vi "Double FFT Mesurament (Max Bin detection - Control - Init Wave&Window - Snapshot) test.vi"() -> ()   [LabVIEW 2014]
uses:
  <vilib>/Platform/TimedLoop/XDataNode/timing_clust.ctl
  <vilib>/Platform/TimedLoop/XDataNode/nitl_modes.ctl
  <vilib>/Platform/TimedLoop/XDataNode/wakeup.ctl
  <vilib>/rvi/Analysis/measure/FFT/simModelSupport/niFPGA FFT Streaming Sim Properties.ctl
  <vilib>/rvi/Analysis/measure/FFT/simModelSupport/niFPGA FFT Sim Stream Group Properties.ctl
  <vilib>/rvi/Analysis/measure/FFT/simModelSupport/niFPGA FFT Sim Types.ctl
  <vilib>/rvi/Analysis/measure/FFT/simModelSupport/niFpgaFFTSimArithmeticProperties.ctl
  <vilib>/rvi/Analysis/measure/FFT/simModelSupport/niFpgaFFTSimDfxp.ctl
  <vilib>/fxp/LVFixedPointQuantizationPolicyTypeDef.ctl
  <vilib>/rvi/Analysis/measure/FFT/XNode/niFpgaFFTButterflyDelays.ctl
  <vilib>/rvi/Emulation/niFpgaSctlEmulationGetInTimedLoop.vi
  <vilib>/rvi/Emulation/niFpgaEmulationReportErrorSimple.vi
  <vilib>/rvi/Emulation/niFpgaGetClockAttributes.vi
  <vilib>/rvi/Emulation/niFpgaCriticalErrorInLSC.vi
  <vilib>/rvi/Emulation/niFpgaEmulationIsFPGAContextNoSignature.vi
  <vilib>/rvi/errors/niFpgaSetErrorForExecOnDevCompSimple.vi
  <vilib>/rvi/eio/common/nirviEmuReportErrorAndStop.vi
  <vilib>/rvi/DataTransferAndStorage/Container/Common/niFpgaContainerGetUniqueNameForEmu.vi
  <vilib>/rvi/FIFO/Fifo_Resource/nirvififoEmulationSetSize.vi
  <vilib>/rvi/FIFO/Fifo_Resource/nirviFifoEmulationQueueMgr.vi
  <instcachedir>/0/nirviFifoEmulationQueueMgr_E5CAEC123FF24DC58D834DCA3CDAA9B5.lvgen/nirviFifoEmulationQueueMgr_E5CAEC123FF24DC58D834DCA3CDAA9B5_012.vi
  <vilib>/rvi/FIFO/Fifo_Resource/nirvififoEmulationCreateLock.vi
  <vilib>/rvi/Emulation/niFpgaProcessEmulError.vi
  <vilib>/rvi/FIFO/Fifo_Resource/nirvififoEmulationObtainLock.vi
  <vilib>/rvi/FIFO/Fifo_Resource/nirvififoEmulationReleaseLock.vi
  <vilib>/rvi/occurrence/nirviWaitOnOccurrenceBase.vi
  <vilib>/rvi/errors/nirviReportUnexpectedCaseInternalError.vi
  <vilib>/rvi/errors/nirviReportUnexpectedCaseInternalError (U32).vi
  <vilib>/rvi/Memory/Memory_Emulation/niFpgaMemoryEmulationCacheClearOnFirstRun.vi
  <vilib>/rvi/Memory/Memory_Emulation/nirvimemoryEmulationManagerCache_MakeExclusive.vi
  <vilib>/rvi/Memory/Memory_Emulation/niFpgaMemoryEmulationValidateCache.vi
  <vilib>/rvi/Memory/Memory_Emulation/nirvimemoryEmulationManagerCache_InsertValue.vi
  <vilib>/Utility/error.llb/Clear Errors.vi
  <vilib>/rvi/Memory/Memory_Emulation/nirvimemoryEmulationManagerCache_ReleaseExclusive.vi
  <vilib>/rvi/Memory/Memory_Emulation/nirvimemoryEmulationManagerCache_GetValue.vi
  <vilib>/rvi/Memory/Memory_Emulation/nirvimemoryEmulationManagerCache_SetValue.vi
  <instcachedir>/0/nirviFifoEmulationQueueMgr_E5CAEC123FF24DC58D834DCA3CDAA9B5.lvgen/nirviFifoEmulationQueueMgr_E5CAEC123FF24DC58D834DCA3CDAA9B5_010.vi
  <vilib>/rvi/FIFO/Fifo_Resource/nirvififoEmulationDetermineInputValidOut.vi
  <vilib>/rvi/Memory/Memory_Emulation/nirvimemoryFastEmulation.vi
  <vilib>/rvi/Memory/Memory_Emulation/nirvimemoryEmulation.vi
  <vilib>/rvi/Analysis/measure/FFT/simModelSupport/niFpgaFFTSimModelStreamingCore.vi
  <vilib>/rvi/interface/RandomDataEmulation/niFpgaRandomDataHandleErrors.vi
  <vilib>/rvi/eio/common/nirviEmuTemplateMethod_errors.vi
  <vilib>/Platform/TimedLoop/XDataNode/XDataNode.xnode
  <vilib>/rvi/DataTransferAndStorage/Container/XNode/niFpgaContainer.xnode
  <vilib>/rvi/FIFO/Fifo_Resource/nirvififoEmulationRead.vi
  <vilib>/rvi/DataTransferAndStorage/Register/Emulation/niFpgaRegisterEmulation.vi
  <vilib>/rvi/FIFO/Fifo_Resource/nirvififoEmulationWrite.vi
  <vilib>/rvi/FIFO/Fifo_Resource/nirvififoEmulationGetNumberOfElementsToWrite.vi
  <vilib>/rvi/Analysis/measure/FFT/XNode/niFpgaFFT.xnode
  <vilib>/rvi/interface/RandomDataEmulation/nirviRandomDataFpgaReadWriteTemplate.vi
  <vilib>/eio/EIOMethodNode/EIOMethodNode.xnode
  <vilib>/Platform/TimedLoop/XDataNode/XDNodeRunTimeDep.lvlib
panel:
  in  "snapshot":bool
  in  "first bin":i32=4
  in  "last bin":i32=251
  in  "lower limit 2":u32=682
  in  "lower limit 1":u32=57
  in  "upper limit 2":u32=1194
  in  "upper limit 1":u32=569
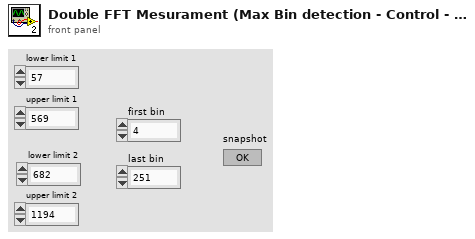
[diagram p1: front panel]
types:
  T1 = typedef "XDNodeRunTimeDep.lvlib/timing_clust.ctl" = cluster{"Expected End [f-1]":u64, "Actual End [f-1]":u64, "Finished Late? [f-1]":bool, "Expected End [i-1]":u64, "Actual End [i-1]":u64, "Finished Late? [i-1]":bool, "Expected Start [i]":u64, "Actual Start [i]":u64, "Expected Start [f]":u64, "Actual Start [f]":u64, "Source Name":string, "Structure Name":string, "Period":i64, "Deadline":i64, "Offset":i64, "Start":i64, "Priority":i32, "Timeout":i32, "Mode":T2, "Wakeup Reason":T3, "Error":errorcluster, "Source Type":string, "Secondary Source Type":string, "Global End Time":u64, "Global Start Time":u64, "Frame Duration":u64, "Iteration Duration":u64, "Assigned CPU":i32, "I/O Scan Engine Mode":u32}
  T2 = typedef "XDNodeRunTimeDep.lvlib/nitl_modes.ctl" = enum32{"No Change", "Process missed periods, maintain original phase", "Discard missed periods, maintain original phase", "Process missed periods, ignore original phase", "Discard missed periods, ignore original phase"}
  T3 = typedef "XDNodeRunTimeDep.lvlib/wakeup.ctl" = enum32{"Normal", "Aborted", "Asynchronous wakeup", "Timing source error", "Timed loop error", "Timeout"}
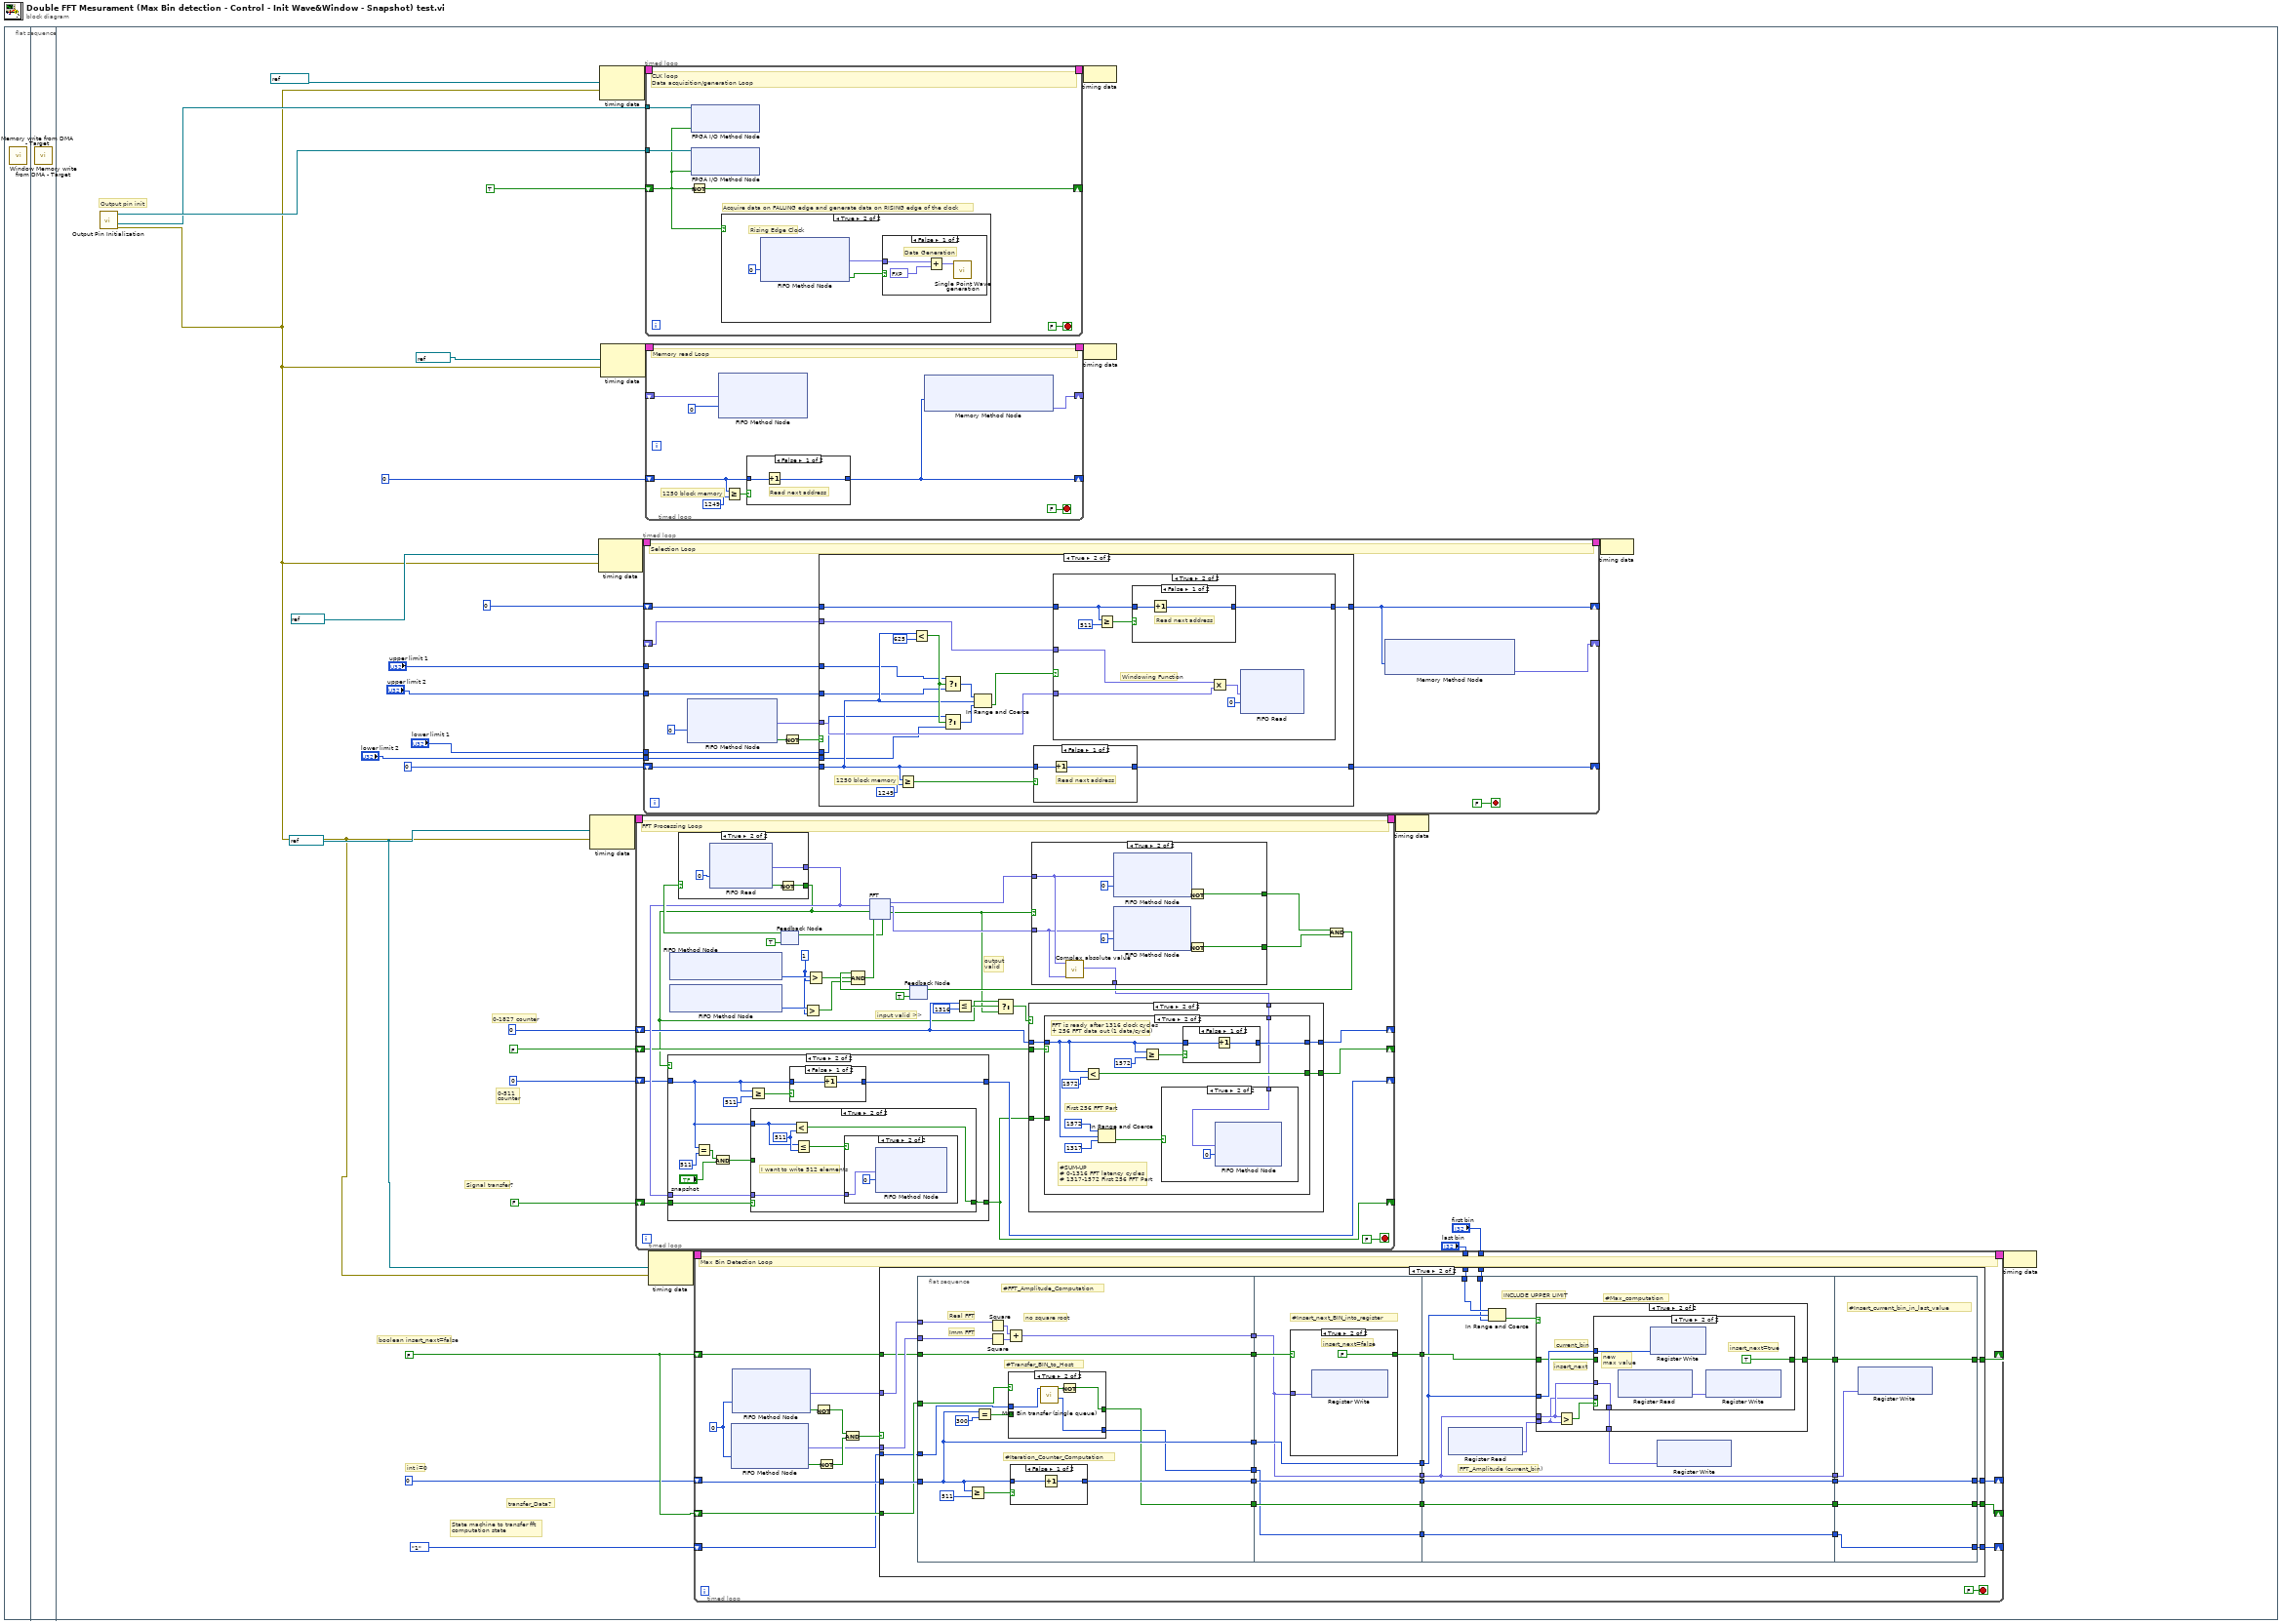
[diagram p0: block diagram]
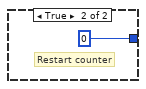
[diagram p4: hidden frame]
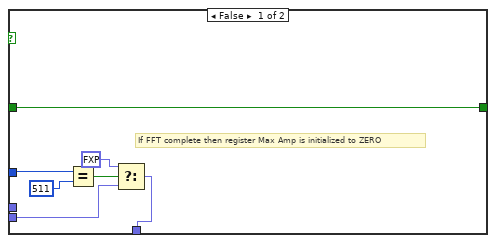
[diagram p6: hidden frame]
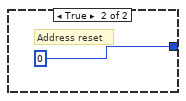
[diagram p10: hidden frame]
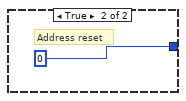
[diagram p11: hidden frame]
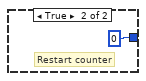
[diagram p15: hidden frame]
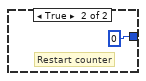
[diagram p19: hidden frame]
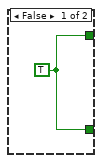
[diagram p20: hidden frame]
diagram:
  n1 = flat-sequence {
    frame #0 {
      n2 = call "Memory write from DMA - Target.vi"() -> ()  [unwired: 12 in]
    }
    frame #1 {
      n3 = call "Window Memory write from DMA - Target.vi"() -> ()  [unwired: 12 in]
    }
    frame #2 {
      w7 = FALSE
      w16 = refnum<k21> "50MHz" ("Source Name")
      # "0-1827 counter"
      # "0-511\ncounter"
      # "Signal transfer?"
      # "State machine to transfer fft\ncomputation state"
      # "transfer_Data?"
      # "int i=0"
      # "boolean insert_next=false"
      # "Output pin init"
      n4 = call "Output Pin Initialization.vi"() -> ("error out"=w15:errorcluster, "I/O Out Clock DAC (pin16)"=w19:refnum<k21>, "I/O Out Clock ADC (pin17)"=w20:refnum<k21>)  [unwired: 8 in]
      n5 = node-c288(w16, w15) -> (w30:T1)
      n6 = node-c288(refnum<k21> "50MHz" ("Source Name"), w15) -> (w28:T1)
      n7 = node-c288(refnum<k21> "100MHz" ("Source Name"), w15) -> (w34:T1)
      n8 = node-c288(refnum<k21> "50MHz" ("Source Name"), w15) -> (w32:T1)
      n9 = timed-loop {
        timing: w30 -> [_]
        timing-out: [_] -> w29
        shift-right: [w232] -> _
        shift-left: FALSE -> [w235]
        shift-right: [w236] -> _
        shift-left: i16 0 -> [w233]
        shift-right: [w231] -> _
        shift-left: FALSE -> [w230]
        shift-right: [w229] -> _
        shift-left: i16 0 -> [w226]
        stop <- FALSE stop-if-true
        w239 = u32 1 ("y")
        # "output\nvalid"
        # "input valid >>"
        # "FFT Processing Loop"
        n10 = xnode ("FIFO Method Node")() -> ("Number of Elements to Write"=w241:u32)  [unwired: 1 in, 1 out]
        n11 = xnode ("FIFO Method Node")() -> ("Number of Elements to Write"=w240:u32)  [unwired: 1 in, 1 out]
        n12 = feedback #1(TRUE ("ready for input")) -> (w253:bool)
        n13 = case shown="True" w253 {
          tunnel: [FALSE w344] -> w224
          tunnel: [fxp<+/-,12,12> 0.0 ("Element") w341] -> w234
          frame False {
            # "RMS is not ready for new input"
          }
          frame True {
            n14 = xnode ("FIFO Read")("Timeout"=0) -> ("Element"=w341:fxp<+/-,12,12>, "Timed Out?"=w343:bool)  [unwired: 1 in, 1 out]
            n15 = Not(x=w343) -> (.not. x?=w344:bool)
          }
        }
        n16 = case shown="True" w224 {
          tunnel: w233 -> [w280 w284]
          tunnel: [w280 w289] -> w236
          tunnel: w235 -> [w279 w282]
          tunnel: [w279 w283] -> w232
          tunnel: w234 -> [_ w281]
          frame False {
          }
          frame True {
            n17 = Equal?(x=w284, y=i16 511) -> (x = y?=w288:bool)
            n18 = And(x=w288, y="snapshot") -> (x .and. y?=w285:bool)
            n19 = Greater Or Equal?(x=w284, y=i16 511) -> (x >= y?=w290:bool)
            n20 = case shown="True" w282 {
              tunnel: w285 -> [w292 _]
              tunnel: w284 -> [_ w293]
              tunnel: [w292 w297] -> w283
              tunnel: w281 -> [_ w295]
              frame False {
              }
              frame True {
                w294 = i16 511 ("y")
                # "I want to write 512 elements"
                n21 = Less?(x=w293, y=w294) -> (x < y?=w297:bool)
                n22 = Less Or Equal?(x=w293, y=w294) -> (x <= y?=w296:bool)
                n23 = case shown="True" w296 {
                  tunnel: w295 -> [_ w298]
                  frame False {
                  }
                  frame True {
                    n24 = xnode ("FIFO Method Node")("Element"=w298, "Timeout"=0) -> ()  [unwired: 1 in, 2 out]
                  }
                }
              }
            }
            n25 = case shown="False" w290 {
              tunnel: w284 -> [w301 _]
              tunnel: [w300 i16 0] -> w289
              frame False {
                n26 = Increment(x=w301) -> (x+1=w300:i16)
              }
              frame True {
                # "Restart counter"
              }
            }
          }
        }
        n27 = Greater?(x=w240, y=w239) -> (0:w237:bool)
        n28 = Greater?(x=w241, y=w239) -> (0:w238:bool)
        n29 = feedback #2(TRUE) -> (w249:bool)
        n30 = Compound Arithmetic op=AND(w249, w238, w237) -> (w248:bool)
        n31 = xnode "FFT"("real data in"=w234, "input valid"=w224, "ready for output"=w248) -> ("ready for input"=w247:bool, "real data out"=w246:fxp<+/-,22,22>, "imaginary data out"=w245:fxp<+/-,22,22>, "output valid"=w222:bool)  [unwired: 2 in, 1 out]
        n32 = feedback-in #1(w247) -> ()
        n33 = Less Or Equal?(x=w226, y=i16 1316) -> (x <= y?=w227:bool)
        n34 = Select(t=w224, s=w227, f=w222) -> (s? t:f=w223:bool)
        n35 = case shown="True" w222 {
          tunnel: w246 -> [_ w332]
          tunnel: w245 -> [_ w331]
          tunnel: [w329 w338] -> w244
          tunnel: [w329 w337] -> w243
          tunnel: [_ w330] -> w228
          frame False {
            w329 = TRUE
          }
          frame True {
            n36 = call "Complex absolute value.vi"("Im"=w331, "Re"=w332) -> ("Square Absolute Value"=w330:fxp<+,44,44>)  [unwired: 9 in]
            n37 = xnode ("FIFO Method Node")("Element"=w332, "Timeout"=0) -> ("Timed Out?"=w333:bool)  [unwired: 1 in, 1 out]
            n38 = xnode ("FIFO Method Node")("Element"=w331, "Timeout"=0) -> ("Timed Out?"=w334:bool)  [unwired: 1 in, 1 out]
            n39 = Not(x=w333) -> (.not. x?=w338:bool)
            n40 = Not(x=w334) -> (.not. x?=w337:bool)
          }
        }
        n41 = case shown="True" w223 {
          tunnel: w232 -> [_ w261]
          tunnel: [w254 w260] -> w231
          tunnel: w230 -> [w254 w259]
          tunnel: w226 -> [w255 w258]
          tunnel: [w255 w257] -> w229
          tunnel: w228 -> [_ w256]
          frame False {
          }
          frame True {
            n42 = case shown="True" w259 {
              tunnel: w261 -> [w263 _]
              tunnel: [w263 w273] -> w260
              tunnel: w258 -> [w262 w266]
              tunnel: [w262 w269] -> w257
              tunnel: w256 -> [_ w264]
              frame False {
              }
              frame True {
                # "First 256 FFT Part"
                # "#SUM-UP\n# 0-1316 FFT latency cycles\n# 1317-1572 First 256 FFT Part"
                # "FFT is ready after 1316 clock cycles\n+ 256 FFT data out (1 data/cycle)"
                n43 = Less?(x=w266, y=i16 1572) -> (x < y?=w273:bool)
                n44 = In Range and Coerce(upper limit=i16 1572, x=w266, lower limit=i16 1317 ("y")) -> (In Range?=w265:bool)  [unwired: 1 out]
                n45 = Greater Or Equal?(x=w266, y=i16 1572) -> (x >= y?=w270:bool)
                n46 = case shown="True" w265 {
                  tunnel: w264 -> [_ w275]
                  frame False {
                  }
                  frame True {
                    n47 = xnode ("FIFO Method Node")("Element"=w275, "Timeout"=0) -> ()  [unwired: 1 in, 2 out]
                  }
                }
                n48 = case shown="False" w270 {
                  tunnel: w266 -> [w277 _]
                  tunnel: [w276 i16 0] -> w269
                  frame False {
                    n49 = Increment(x=w277) -> (x+1=w276:i16)
                  }
                  frame True {
                    # "Restart counter"
                  }
                }
              }
            }
          }
        }
        n50 = Compound Arithmetic op=AND(w244, w243) -> (w242:bool)
        n51 = feedback-in #2(w242) -> ()
      }
      n52 = timed-loop {
        timing: w28 -> [_]
        timing-out: [_] -> w27
        shift-right: [w179] -> _
        shift-left: u32 0 -> [w178]
        tunnel: "upper limit 1" -> [w173]
        tunnel: "upper limit 2" -> [w172]
        tunnel: "lower limit 1" -> [w171]
        tunnel: "lower limit 2" -> [w170]
        shift-right: [w166] -> _
        shift-left: u32 0 -> [w169]
        shift-right: [w167] -> _
        shift-left: _ -> [w168]
        stop <- FALSE stop-if-true
        # "Selection Loop"
        n53 = xnode ("FIFO Method Node")("Timeout"=0) -> ("Element"=w175:fxp<+/-,12,12>, "Timed Out?"=w176:bool)  [unwired: 1 in, 1 out]
        n54 = Not(x=w176) -> (.not. x?=w177:bool)
        n55 = case shown="True" w177 {
          tunnel: [w182 w197] -> w179
          tunnel: w178 -> [w182 w192]
          tunnel: w175 -> [_ w190]
          tunnel: w173 -> [_ w189]
          tunnel: w172 -> [_ w188]
          tunnel: w171 -> [_ w187]
          tunnel: w170 -> [_ w186]
          tunnel: w169 -> [w181 w183]
          tunnel: [w181 w185] -> w166
          tunnel: w168 -> [_ w184]
          frame False {
          }
          frame True {
            # "1250 block memory"
            n56 = Greater Or Equal?(x=w192, y=u32 1249) -> (x >= y?=w198:bool)
            n57 = Less?(x=w192, y=u32 625) -> (x < y?=w193:bool)
            n58 = Select(t=w187, s=w193, f=w186) -> (s? t:f=w195:u32)
            n59 = Select(t=w189, s=w193, f=w188) -> (s? t:f=w196:u32)
            n60 = In Range and Coerce(upper limit=w196, x=w192, lower limit=w195) -> (In Range?=w191:bool)  [unwired: 1 out]
            n61 = case shown="False" w198 {
              tunnel: w192 -> [w213 _]
              tunnel: [w212 u32 0] -> w197
              frame False {
                # "Read next address"
                n62 = Increment(x=w213) -> (x+1=w212:u32)
              }
              frame True {
                # "Address reset"
              }
            }
            n63 = case shown="True" w191 {
              tunnel: w190 -> [_ w201]
              tunnel: w183 -> [w200 w206]
              tunnel: [w200 w208] -> w185
              tunnel: w184 -> [_ w204]
              frame False {
              }
              frame True {
                # "Windowing Function"
                n64 = Greater Or Equal?(x=w206, y=u32 511) -> (x >= y?=w207:bool)
                n65 = case shown="False" w207 {
                  tunnel: w206 -> [w210 _]
                  tunnel: [w209 u32 0] -> w208
                  frame False {
                    # "Read next address"
                    n66 = Increment(x=w210) -> (x+1=w209:u32)
                  }
                  frame True {
                    # "Address reset"
                  }
                }
                n67 = Multiply(x=w204, y=w201) -> (x*y=w202:fxp<+/-,12,12>)
                n68 = xnode ("FIFO Read")("Element"=w202, "Timeout"=0) -> ()  [unwired: 1 in, 2 out]
              }
            }
          }
        }
        n69 = xnode ("Memory Method Node")("Address"=w166) -> ("Data"=w167:fxp<+,8,1>)  [unwired: 1 in, 1 out]
      }
      n70 = timed-loop {
        timing: w34 -> [_]
        timing-out: [_] -> w33
        shift-right: [w372] -> _
        shift-left: TRUE -> [w370]
        tunnel: w19 -> [w374]
        tunnel: w20 -> [w371]
        stop <- FALSE stop-if-true
        # "Acquire data on FALLING edge and generate data on RISING edge of the clock"
        # "CLK loop\nData acquisition/generation Loop"
        n71 = Not(x=w370) -> (.not. x?=w372:bool)
        n72 = xnode "FPGA I/O Method Node"("FPGA I/O In"=w374, "Data"=w370) -> ()  [unwired: 1 out]
        n73 = xnode "FPGA I/O Method Node"("FPGA I/O In"=w371, "Data"=w370) -> ()  [unwired: 1 out]
        n74 = case shown="True" w370 {
          frame False {
            # "Falling Edge Clock"
            n75 = call "Single Acquisition.vi"() -> ("Out"=w376:fxp<+/-,12,12>)  [unwired: 10 in, 1 out]
            n76 = xnode ("FIFO Method Node")("Element"=w376, "Timeout"=0) -> ()  [unwired: 1 in, 2 out]
          }
          frame True {
            # "Rising Edge Clock"
            n77 = xnode ("FIFO Method Node")("Timeout"=0) -> ("Element"=w377:fxp<+/-,12,12>, "Timed Out?"=w378:bool)  [unwired: 1 in, 1 out]
            n78 = case shown="False" w378 {
              tunnel: w377 -> [w382 _]
              frame False {
                # "Data Generation"
                n79 = Add(x=w382, y=fxp<+,12,12> 2048.0) -> (x+y=w380:fxp<+/-,14,14>)
                n80 = call "Single Point Wave generation.vi"("Data To Write"=w380) -> ()  [unwired: 10 in, 1 out]
              }
              frame True {
                # "FPGA memory slow"
              }
            }
          }
        }
      }
      n81 = timed-loop {
        timing: w32 -> [_]
        timing-out: [_] -> w31
        shift-right: [w352] -> _
        shift-left: u32 0 -> [w356]
        shift-right: [w354] -> _
        shift-left: _ -> [w353]
        stop <- FALSE stop-if-true
        # "1250 block memory"
        # "Memory read Loop"
        n82 = xnode ("FIFO Method Node")("Element"=w353, "Timeout"=0) -> ()  [unwired: 1 in, 2 out]
        n83 = Greater Or Equal?(x=w356, y=u32 1249) -> (x >= y?=w358:bool)
        n84 = case shown="False" w358 {
          tunnel: w356 -> [w361 _]
          tunnel: [w360 u32 0] -> w352
          frame False {
            # "Read next address"
            n85 = Increment(x=w361) -> (x+1=w360:u32)
          }
          frame True {
            # "Address reset"
          }
        }
        n86 = xnode ("Memory Method Node")("Address"=w352) -> ("Data"=w354:fxp<+/-,12,12>)  [unwired: 1 in, 1 out]
      }
      n87 = node-c288(w16, w15) -> (w26:T1)
      n88 = timed-loop {
        shift-right: [w45] -> _
        shift-left: 0 ("Timeout") -> [w46]
        shift-right: [w43] -> _
        shift-left: w7 -> [w44]
        timing: w26 -> [_]
        timing-out: [_] -> w25
        tunnel: "last bin" -> [w41]
        tunnel: "first bin" -> [w40]
        shift-right: [w37] -> _
        shift-left: w7 -> [w38]
        shift-right: [w35] -> _
        shift-left: enum16{"1", "2", "3", "4"}."1" ("Enum") -> [w36]
        stop <- FALSE stop-if-true
        w39 = 0 ("Timeout")
        # "Max Bin Detection Loop"
        n89 = xnode ("FIFO Method Node")("Timeout"=w39) -> ("Element"=w47:fxp<+/-,22,22>, "Timed Out?"=w52:bool)  [unwired: 1 in, 1 out]
        n90 = xnode ("FIFO Method Node")("Timeout"=w39) -> ("Element"=w48:fxp<+/-,22,22>, "Timed Out?"=w53:bool)  [unwired: 1 in, 1 out]
        n91 = Not(x=w53) -> (.not. x?=w51:bool)
        n92 = Not(x=w52) -> (.not. x?=w50:bool)
        n93 = And(x=w51, y=w50) -> (x .and. y?=w49:bool)
        n94 = case shown="True" w49 {
          tunnel: w48 -> [_ w86]
          tunnel: w47 -> [_ w85]
          tunnel: w46 -> [w57 w83]
          tunnel: [w57 w70] -> w45
          tunnel: w44 -> [w56 w77]
          tunnel: [w56 w72] -> w43
          tunnel: w41 -> [_ w69]
          tunnel: w40 -> [_ w68]
          tunnel: w38 -> [w55 w67]
          tunnel: [w55 w66] -> w37
          tunnel: w36 -> [w54 w62]
          tunnel: [w54 w58] -> w35
          frame False {
            # "Data are NOT ready in Target Real FFT and Target Imm FFT FIFOs"
          }
          frame True {
            n95 = flat-sequence {
              tunnel: w86 -> [w99]
              tunnel: w85 -> [w100]
              tunnel: [w93] -> w84
              tunnel: w83 -> [w92]
              tunnel: [w98] -> w82
              tunnel: [w92] -> w79
              tunnel: [w95] -> w78
              tunnel: w77 -> [w95]
              tunnel: w67 -> [w91]
              tunnel: [w89] -> w65
              tunnel: w62 -> [w88]
              tunnel: [w87] -> w59
              tunnel: w84 -> [w115]
              tunnel: w82 -> [w118]
              tunnel: [w118] -> w81
              tunnel: w79 -> [w116]
              tunnel: w78 -> [w117]
              tunnel: [w116] -> w76
              tunnel: [w115] -> w75
              tunnel: [w114] -> w74
              tunnel: w65 -> [w113]
              tunnel: [w113] -> w64
              tunnel: [w112] -> w60
              tunnel: w59 -> [w112]
              tunnel: w81 -> [w133]
              tunnel: [w133] -> w80
              tunnel: w76 -> [w128]
              tunnel: w75 -> [w130]
              tunnel: w74 -> [w131]
              tunnel: [w130] -> w73
              tunnel: [w129] -> w71
              tunnel: w69 -> [w125]
              tunnel: w68 -> [w124]
              tunnel: w64 -> [w123]
              tunnel: [w123] -> w63
              tunnel: [w122] -> w61
              tunnel: w60 -> [w122]
              tunnel: w80 -> [w156]
              tunnel: w73 -> [w158]
              tunnel: w71 -> [w157]
              tunnel: [w157] -> w72
              tunnel: [w156] -> w70
              tunnel: [w155] -> w66
              tunnel: w63 -> [w155]
              tunnel: w61 -> [w154]
              tunnel: [w154] -> w58
              frame #0 {
                # "no square root"
                # "#Transfer_BIN_to_Host"
                # "#Iteration_Counter_Computation"
                # "#FFT_Amplitude_Computation"
                # "Imm FFT"
                # "Real FFT"
                n96 = Greater Or Equal?(x=w92, y=511) -> (x >= y?=w96:bool)
                n97 = Equal?(x=w92, y=300) -> (x = y?=w90:bool)
                n98 = Square(x=w99) -> (x^2=w102:fxp<+,43,43>)
                n99 = Square(x=w100) -> (x^2=w101:fxp<+,43,43>)
                n100 = Add(x=w102, y=w101) -> (x+y=w93:fxp<+,44,44>)
                n101 = case shown="True" w91 {
                  tunnel: w90 -> [w104 _]
                  tunnel: [w104 w107] -> w89
                  tunnel: w88 -> [w103 w106]
                  tunnel: [w103 w105] -> w87
                  frame False {
                    # "FFT Comp is NOT finished"
                  }
                  frame True {
                    n102 = call "Max Bin transfer (single queue).vi"("Enum"=w106) -> ("Next state"=w105:enum16{"1", "2", "3", "4"}, "END?"=w108:bool)  [unwired: 9 in]
                    n103 = Not(x=w108) -> (.not. x?=w107:bool)
                  }
                }
                n104 = case shown="False" w96 {
                  tunnel: w92 -> [w109 _]
                  tunnel: [w110 0 ("Timeout")] -> w98
                  frame False {
                    n105 = Increment(x=w109) -> (x+1=w110:i32)
                  }
                  frame True {
                    # "Restart counter"
                  }
                }
              }
              frame #1 {
                # "#Insert_next_BIN_into_register"
                n106 = case shown="True" w117 {
                  selector: w117 -> [w119 _]
                  tunnel: [w119 FALSE] -> w114
                  tunnel: w115 -> [_ w120]
                  frame False {
                  }
                  frame True {
                    # "insert_next=false"
                    n107 = xnode ("Register Write")("Data"=w120) -> ()  [unwired: 1 in, 1 out]
                  }
                }
              }
              frame #2 {
                # "INCLUDE UPPER LIMIT"
                # "FFT_Amplitude (current_bin)"
                # "#Max_computation"
                n108 = xnode ("Register Read")() -> ("Data"=w127:fxp<+,44,44>)  [unwired: 1 in, 1 out]
                n109 = In Range and Coerce(upper limit=w125, x=w128, lower limit=w124) -> (In Range?=w132:bool)  [unwired: 1 out]
                n110 = case shown="True" w132 {
                  tunnel: w130 -> [_ w146]
                  tunnel: w128 -> [w138 w145]
                  tunnel: w131 -> [w140 w144]
                  tunnel: [w140 w143] -> w129
                  tunnel: w127 -> [w136 w141]
                  tunnel: [w134 w142] -> w126
                  frame False {
                    # "If FFT complete then register Max Amp is initialized to ZERO"
                    n111 = Equal?(x=w138, y=511) -> (x = y?=w139:bool)
                    n112 = Select(t=fxp<+,44,44> 0.0, s=w139, f=w136) -> (s? t:f=w134:fxp<+,44,44>)
                  }
                  frame True {
                    # "insert_next"
                    # "current_bin"
                    n113 = Greater?(x=w146, y=w141) -> (0:w147:bool)
                    n114 = case shown="True" w147 {
                      tunnel: w146 -> [_ w150]
                      tunnel: w145 -> [_ w153]
                      tunnel: w144 -> [w149 _]
                      tunnel: [w149 TRUE] -> w143
                      tunnel: [w148 w150] -> w142
                      tunnel: w141 -> [w148 _]
                      frame False {
                        # "Old value is re-written"
                      }
                      frame True {
                        # "new\nmax value"
                        # "insert_next=true"
                        n115 = xnode ("Register Read")() -> ("Data"=w151:fxp<+,44,44>)  [unwired: 1 in, 1 out]
                        n116 = xnode ("Register Write")("Data"=w153) -> ()  [unwired: 1 in, 1 out]
                        n117 = xnode ("Register Write")("Data"=w151) -> ()  [unwired: 1 in, 1 out]
                      }
                    }
                  }
                }
                n118 = xnode ("Register Write")("Data"=w126) -> ()  [unwired: 1 in, 1 out]
              }
              frame #3 {
                # "#Insert_current_bin_in_last_value"
                n119 = xnode ("Register Write")("Data"=w158) -> ()  [unwired: 1 in, 1 out]
              }
            }
          }
        }
      }
      n120 = node-c288(w33) -> ()
      n121 = node-c288(w31) -> ()
      n122 = node-c288(w29) -> ()
      n123 = node-c288(w27) -> ()
      n124 = node-c288(w25) -> ()
    }
  }
